vi "Digital Static In.vi"() -> ()   [LabVIEW 2018]
uses:
  Submodules/Source/Types/Static.Measure.Digital.Measurement.ctl
  <vilib>/rvi/Emulation/niFpgaGetClockAttributes.vi
  <vilib>/rvi/Emulation/niFpgaSctlEmulationGetInTimedLoop.vi
  <vilib>/rvi/Emulation/niFpgaEmulationReportErrorSimple.vi
  <vilib>/rvi/Emulation/niFpgaCriticalErrorInLSC.vi
  Submodules/Source/Speciality FPGA IO.lvlib
panel:
  in  "STATE":bool
  out "Digital Static In":T1
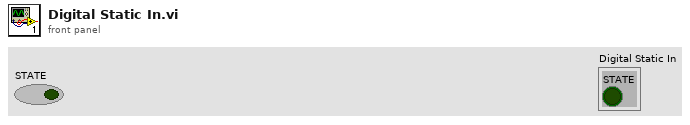
[diagram p1: front panel]
types:
  T1 = typedef "Speciality FPGA IO.lvlib/Static.Measure.Digital.Measurement.ctl" = cluster{"STATE":bool}
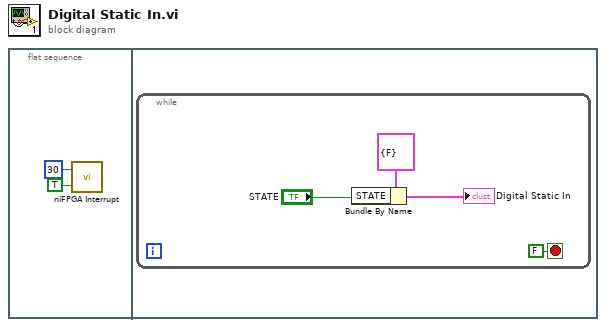
[diagram p0: block diagram]
diagram:
  n1 = flat-sequence {
    frame #0 {
      n2 = call <vilib>:"niFPGA Interrupt.vi"("Wait Until Cleared (F)"=TRUE, "IRQ Number (0)"=u8 30) -> ()  [unwired: 1 in]
    }
    frame #1 {
      n3 = while {
        stop <- FALSE stop-if-true
        n4 = Bundle By Name(cluster=T1 {"STATE"=FALSE}, "STATE"="STATE") -> (→"Digital Static In":T1)
      }
    }
  }
